vi "SPIM control3d-PID.vi"() -> ()   [LabVIEW 2012]
uses:
  Scanning Setting.vi
panel:
  in  "1 Slice":bool
  in  "Structual":bool
  in  "Funcational":bool
  out "Peizo Voltage":dbl
  out "Peizo Location":dbl
  out "Z-Offset":dbl
  out "Scan Signal 2":cluster{"Y":dbl[], "Y":dbl[]}[](graph)
  out "Trigger":dynamicdata(graph)=[{"t0"=timestamp(16448.7 s since 1904-01-01), "dt"=1e-05, "Y"=array[10000 elements], "attributes"=variant("NI_ChannelName"=variant(string "Triangle (Collected)"), "NI_ExpIsRelativeTime"=variant(bool TRUE), "NI_ExpStartTimeStamp"=variant(timestamp timestamp(3461934223.089551 s since 1904-01-01)), "NI_ExpTimeStamp"=variant(timestamp timestamp(3461934223.089551 s since 1904-01-01)), "NI_ExpXDimension"=variant(string "t"), "NI_OriginalChannelName"=variant(string "Triangle"))}, {"t0"=timestamp(16448.7 s since 1904-01-01), "dt"=1e-05, "Y"=array[10000 elements], "attributes"=variant("NI_ChannelName"=variant(string "Square (Collected)"), "NI_ExpIsRelativeTime"=variant(bool TRUE), "NI_ExpStartTimeStamp"=variant(timestamp timestamp(3461934223.089551 s since 1904-01-01)), "NI_ExpTimeStamp"=variant(timestamp timestamp(3461934223.089551 s since 1904-01-01)), "NI_ExpXDimension"=variant(string "t"), "NI_OriginalChannelName"=variant(string "Square"))}, {"t0"=timestamp(16448.7 s since 1904-01-01), "dt"=1e-05, "Y"=array[10000 elements], "attributes"=variant("NI_ChannelName"=variant(string "Square (Collected)"), "NI_ExpIsRelativeTime"=variant(bool TRUE), "NI_ExpStartTimeStamp"=variant(timestamp timestamp(3461934223.0885506 s since 1904-01-01)), "NI_ExpTimeStamp"=variant(timestamp timestamp(3461934223.0885506 s since 1904-01-01)), "NI_ExpXDimension"=variant(string "t"), "NI_OriginalChannelName"=variant(string "Square"))}]
  out "Scan Signal":cluster{"Y":dbl[], "Y":dbl[]}[](graph)
  out "Error Out":errorcluster={"status"=TRUE, "code"=-200561, "source"="SPIM control.vi:Instance:14:1<append>\n<B>Data: </B>-10.007205\n<B>Specified Range Minimum: </B>-10.0\n<B>Specified Range Maximum: </B> 10.0\n\n<B>Task Name: </B>_unnamedTask<30>"}
  in  "Scanner":bool
  in  "Setting":bool
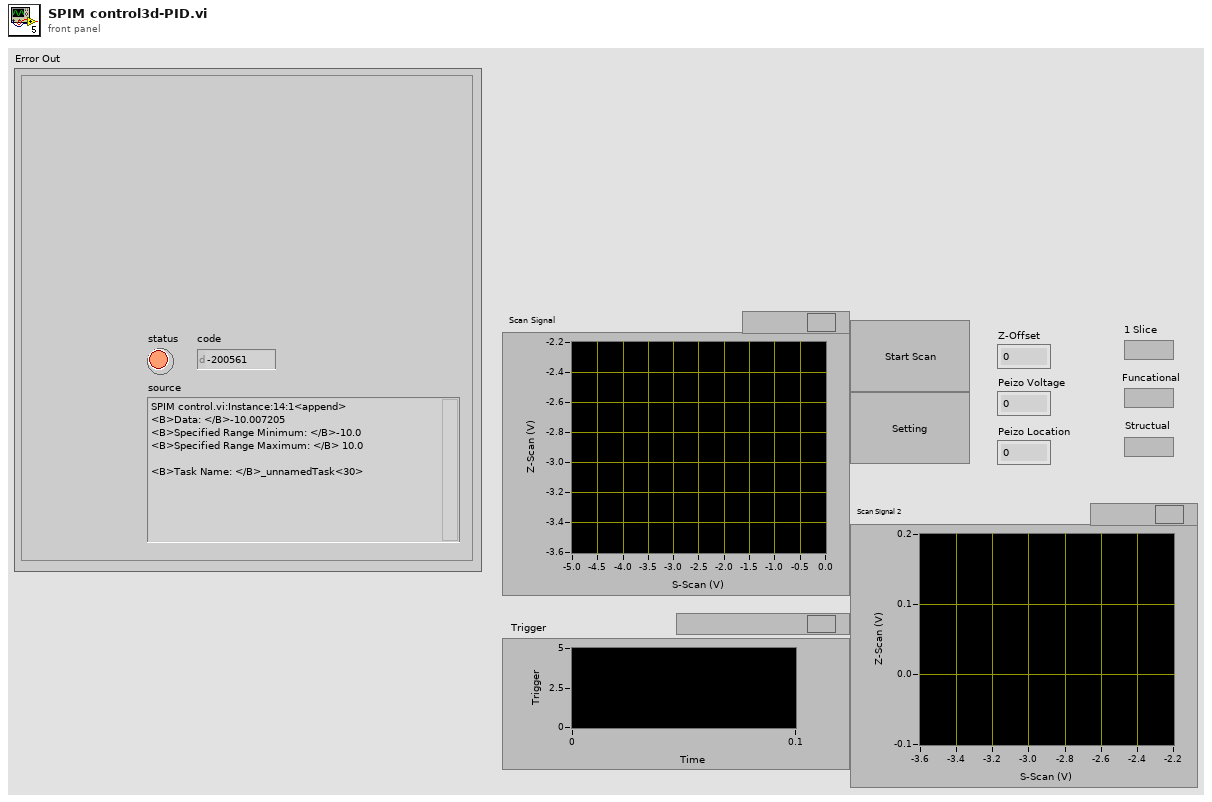
[diagram p1: front panel]
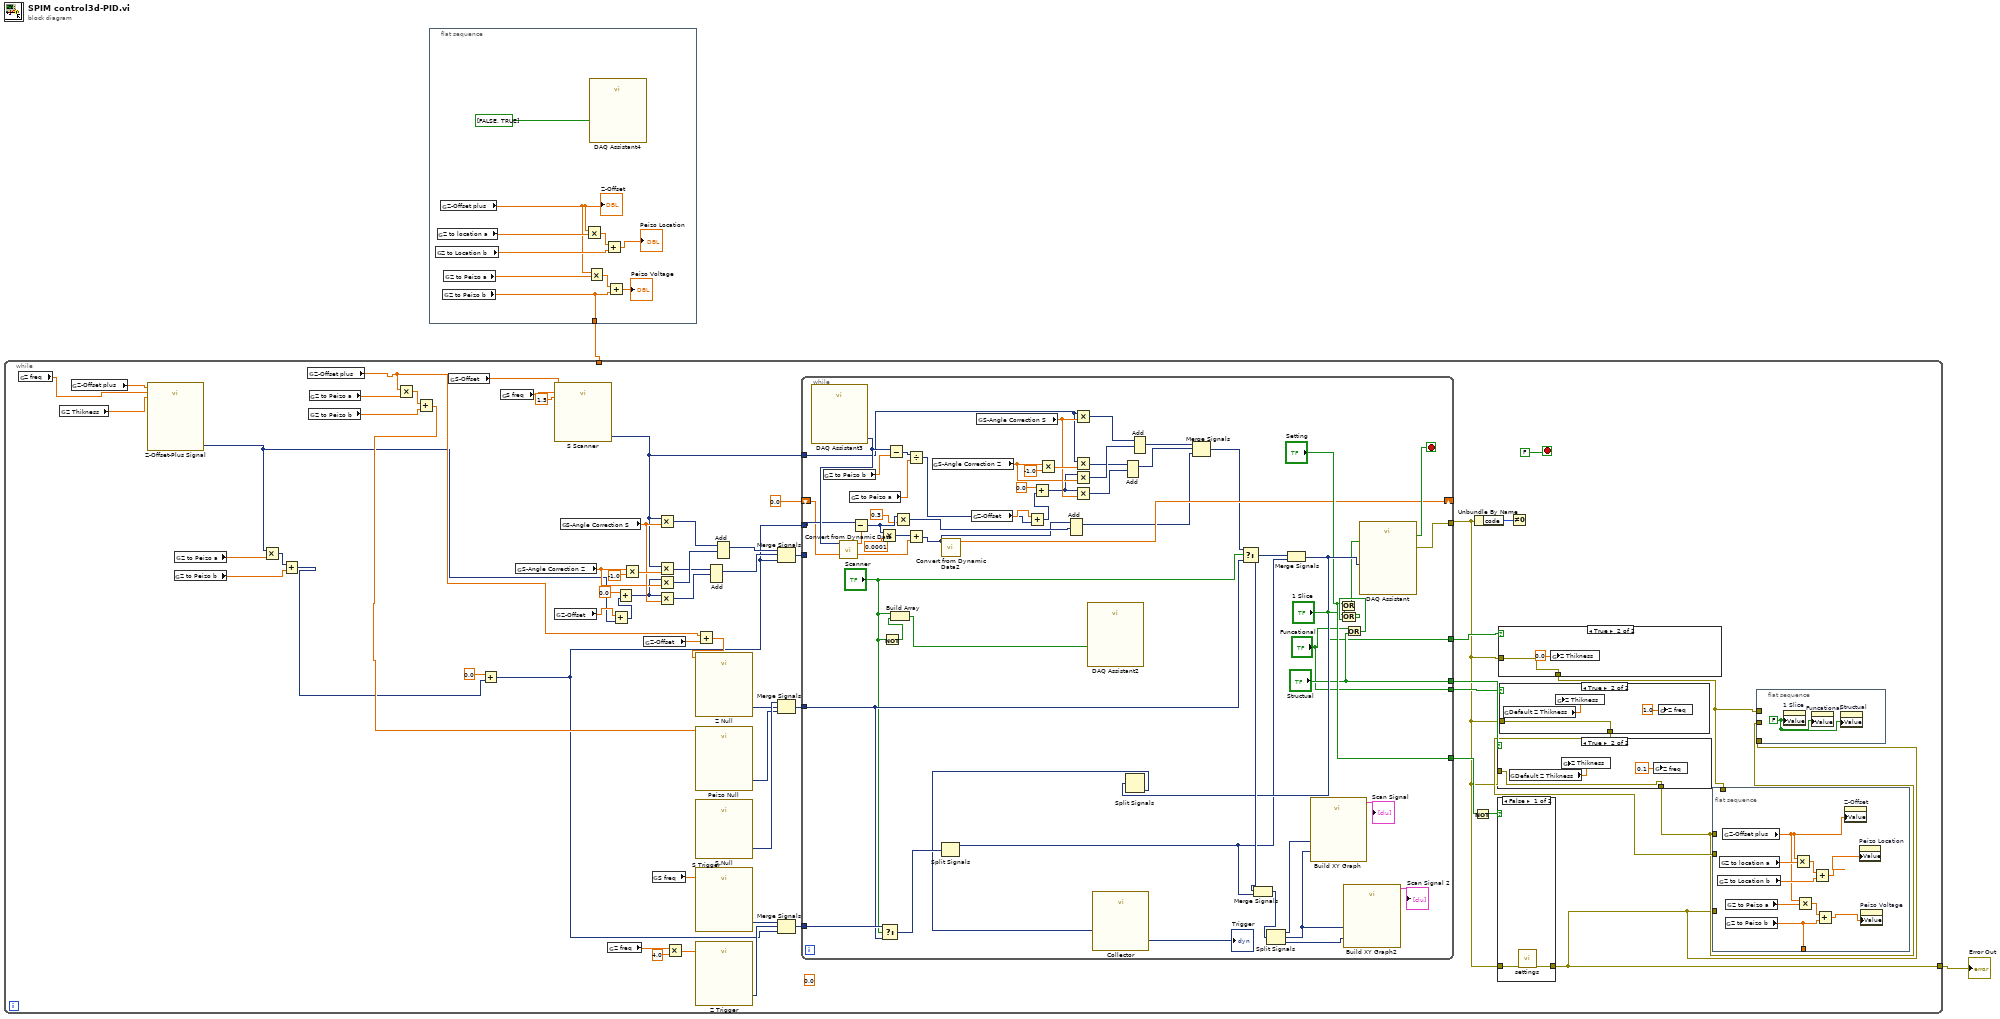
[diagram p0: block diagram]
diagram:
  n1 = while {
    tunnel: [w10] -> w1
    tunnel: w2 -> [_]
    stop <- FALSE stop-if-true
    (unwired) 0.0 ("Offset")
    n2 = global read "Scanning Setting.vi" "Z freq"() -> (w19:dbl)
    n3 = global read "Scanning Setting.vi" "Z Thikness"() -> (w20:dbl)
    n4 = global read "Scanning Setting.vi" "Z-Offset plus"() -> (w26:dbl)
    n5 = call "Z-Offset-Plus Signal"("Offset"=w26, "Frequency"=w19, "Amplitude"=w20) -> ("Triangle"=w21:dynamicdata)  [unwired: 11 in, 1 out]
    n6 = global read "Scanning Setting.vi" "Z to Peizo b"() -> (w25:dbl)
    n7 = global read "Scanning Setting.vi" "Z to Peizo a"() -> (w24:dbl)
    n8 = Multiply(x=w21, y=w24) -> (x*y=w23:dynamicdata)
    n9 = Add(x=w23, y=w25) -> (x+y=w22:dynamicdata)
    n10 = global read "Scanning Setting.vi" "Z-Offset plus"() -> (w27:dbl)
    n11 = global read "Scanning Setting.vi" "Z to Peizo b"() -> (w29:dbl)
    n12 = global read "Scanning Setting.vi" "Z to Peizo a"() -> (w30:dbl)
    n13 = Multiply(x=w27, y=w30) -> (x*y=w31:dbl)
    n14 = Add(x=w31, y=w29) -> (x+y=w28:dbl)
    n15 = global read "Scanning Setting.vi" "S-Offset"() -> (w50:dbl)
    n16 = Add(x=0.0, y=w22) -> (x+y=w5:dynamicdata)
    n17 = global read "Scanning Setting.vi" "S freq"() -> (w51:dbl)
    n18 = global read "Scanning Setting.vi" "S-Angle Correction Z"() -> (w48:dbl)
    n19 = call "S Scanner"("Offset"=w50, "Frequency"=w51, "Amplitude"=1.5) -> ("Triangle"=w6:dynamicdata)  [unwired: 11 in, 1 out]
    n20 = global read "Scanning Setting.vi" "Z-Offset"() -> (w35:dbl)
    n21 = global read "Scanning Setting.vi" "S-Angle Correction S"() -> (w49:dbl)
    n22 = global read "Scanning Setting.vi" "Z freq"() -> (w39:dbl)
    n23 = Add(x=w35, y=w21) -> (x+y=w34:dynamicdata)
    n24 = Add(x=0.0, y=w34) -> (x+y=w37:dynamicdata)
    n25 = Multiply(x=w48, y=-1.0) -> (x*y=w54:dbl)
    n26 = global read "Scanning Setting.vi" "Z-Offset"() -> (w33:dbl)
    n27 = global read "Scanning Setting.vi" "S freq"() -> (w45:dbl)
    n28 = Multiply(x=w6, y=w49) -> (x*y=w57:dynamicdata)
    n29 = Multiply(x=w6, y=w54) -> (x*y=w55:dynamicdata)
    n30 = Multiply(x=w37, y=w48) -> (x*y=w58:dynamicdata)
    n31 = Multiply(x=w37, y=w49) -> (x*y=w56:dynamicdata)
    n32 = Multiply(x=w39, y=4.0) -> (x*y=w40:dbl)
    n33 = call "Peizo Null"("Offset"=w28) -> ("Square"=w36:dynamicdata)  [unwired: 13 in, 1 out]
    n34 = call "S Null"() -> ("Triangle"=w62:dynamicdata)  [unwired: 14 in, 1 out]
    n35 = call "S Trigger"("Frequency"=w45) -> ("Square"=w44:dynamicdata)  [unwired: 13 in, 1 out]
    n36 = call "Z Trigger"("Frequency"=w40) -> ("Square"=w43:dynamicdata)  [unwired: 13 in, 1 out]
    n37 = Add(x=w27, y=w33) -> (x+y=w32:dbl)
    n38 = call "Z Null"("Offset"=w32) -> ("Square"=w47:dynamicdata)  [unwired: 13 in, 1 out]
    n39 = Add(1:w56, 2:w55) -> (0:w52:dynamicdata)  [unwired: 1 in, 1 out]
    n40 = Add(1:w58, 2:w57) -> (0:w46:dynamicdata)  [unwired: 1 in, 1 out]
    n41 = Merge Signals(w46, w52, w5) -> (w61:dynamicdata)
    n42 = Merge Signals(w62, w47, w36) -> (w60:dynamicdata)
    n43 = Merge Signals(w44, w43, w5) -> (w42:dynamicdata)
    n44 = while {
      tunnel: w61 -> [_]
      tunnel: w60 -> [w138]
      tunnel: [w142] -> w9
      tunnel: w42 -> [w139]
      tunnel: ["Setting"] -> w17
      tunnel: ["Structual"] -> w16
      tunnel: ["Funcational"] -> w15
      tunnel: ["1 Slice"] -> w14
      tunnel: w6 -> [w87]
      tunnel: w5 -> [w99]
      shift-right: [w94] -> _
      shift-left: 0.0 ("x") -> [w95]
      stop <- w144 stop-if-true
      n45 = call "DAQ Assistant3"() -> ("data"=w100:dynamicdata)  [unwired: 16 in, 3 out]
      n46 = global read "Scanning Setting.vi" "Z to Peizo b"() -> (w118:dbl)
      n47 = call "Convert from Dynamic Data"("Dynamic Data Type"=w100) -> ("Scalar"=w98:dbl)  [unwired: 3 in]
      n48 = global read "Scanning Setting.vi" "Z to Peizo a"() -> (w116:dbl)
      n49 = Subtract(x=w99, y=w98) -> (x-y=w93:dynamicdata)
      n50 = Multiply(x=w93, y=0.0001) -> (x*y=w96:dynamicdata)
      n51 = Select(t=w139, s="Scanner", f=w138) -> (s? t:f=w133:dynamicdata)
      n52 = Not(x="Scanner") -> (.not. x?=w120:bool)
      n53 = Subtract(x=w100, y=w118) -> (x-y=w117:dynamicdata)
      n54 = Build Array("Scanner", w120) -> (w121:bool[])
      n55 = Multiply(x=w93, y=0.3) -> (x*y=w91:dynamicdata)
      n56 = Divide(x=w117, y=w116) -> (x/y=w103:dynamicdata)
      n57 = Add(x=w96, y=w95) -> (x+y=w90:dynamicdata)
      n58 = global read "Scanning Setting.vi" "S-Angle Correction Z"() -> (w108:dbl)
      n59 = Split Signals(w133) -> (w129:dynamicdata)  [unwired: 3 in, 2 out]
      n60 = call "Convert from Dynamic Data2"("Dynamic Data Type"=w90) -> ("Scalar"=w94:dbl)  [unwired: 3 in]
      n61 = global read "Scanning Setting.vi" "Z-Offset"() -> (w106:dbl)
      n62 = global read "Scanning Setting.vi" "S-Angle Correction S"() -> (w109:dbl)
      n63 = Add(x=w106, y=w103) -> (x+y=w105:dynamicdata)
      n64 = Add(x=0.0, y=w105) -> (x+y=w107:dynamicdata)
      n65 = Multiply(x=w108, y=-1.0) -> (x*y=w111:dbl)
      n66 = Add(1:w91, 2:w90) -> (0:w89:dynamicdata)  [unwired: 1 in, 1 out]
      n67 = Multiply(x=w87, y=w109) -> (x*y=w114:dynamicdata)
      n68 = Multiply(x=w87, y=w111) -> (x*y=w112:dynamicdata)
      n69 = Multiply(x=w107, y=w108) -> (x*y=w115:dynamicdata)
      n70 = Multiply(x=w107, y=w109) -> (x*y=w113:dynamicdata)
      n71 = call "DAQ Assistant2"("data"=w121) -> ()  [unwired: 17 in, 2 out]
      n72 = Add(1:w113, 2:w112) -> (0:w101:dynamicdata)  [unwired: 1 in, 1 out]
      n73 = Add(1:w115, 2:w114) -> (0:w102:dynamicdata)  [unwired: 1 in, 1 out]
      n74 = Merge Signals(w102, w101, w89) -> (w88:dynamicdata)
      n75 = Select(t=w88, s="Scanner", f=w138) -> (s? t:f=w141:dynamicdata)
      n76 = Merge Signals(w141, w129) -> (w130:dynamicdata)
      n77 = Split Signals(w130) -> (w135:dynamicdata, w136:dynamicdata, w134:dynamicdata)  [unwired: 3 in]
      n78 = Merge Signals(w141, w129) -> (w132:dynamicdata)
      n79 = Split Signals(w132) -> (w131:dynamicdata)  [unwired: 4 in, 3 out]
      n80 = call "Collector"("Signals"=w131) -> ("Collected Signals"=→"Trigger":dynamicdata)  [unwired: 9 in, 1 out]
      n81 = call "Build XY Graph"("Y Input"=w136, "X Input"=w135) -> ("XY Graph"=→"Scan Signal":cluster{"Y":dbl[], "Y":dbl[]}[])  [unwired: 3 in, 6 out]
      n82 = call "Build XY Graph2"("Y Input"=w134, "X Input"=w136) -> ("XY Graph"=→"Scan Signal 2":cluster{"Y":dbl[], "Y":dbl[]}[])  [unwired: 3 in, 6 out]
      n83 = Or(x="Funcational", y="Structual") -> (x .or. y?=w128:bool)
      n84 = Or(x="1 Slice", y=w128) -> (x .or. y?=w127:bool)
      n85 = Or(x="Setting", y=w127) -> (x .or. y?=w125:bool)
      n86 = call "DAQ Assistant"("data"=w132, "stop (F)"=w125) -> ("stopped"=w144:bool, "error out"=w142:errorcluster)  [unwired: 15 in, 1 out]
    }
    n87 = Not(x=w17) -> (.not. x?=w18:bool)
    n88 = Unbundle By Name(w9) -> ("code"=w38:i32)
    n89 = case shown="True" w16 {
      tunnel: w9 -> [w71 w72]
      tunnel: [w71 w72] -> w11
      frame False {
      }
      frame True {
        n90 = global read "Scanning Setting.vi" "Default Z Thikness"() -> (w74:dbl)
        n91 = global write "Scanning Setting.vi" "Z Thikness"(w74) -> ()
        n92 = global write "Scanning Setting.vi" "Z freq"(0.1 ("Z freq")) -> ()
      }
    }
    n93 = case shown="False" w18 {
      tunnel: [w84 w86] -> w10
      tunnel: w9 -> [w85 w86]
      frame False {
        n94 = call "settings.vi"("Error In"=w85) -> ("Error Out"=w84:errorcluster)  [unwired: 10 in]
      }
      frame True {
      }
    }
    n95 = case shown="True" w14 {
      tunnel: w9 -> [w64 w65]
      tunnel: [w64 w65] -> w12
      frame False {
      }
      frame True {
        n96 = global write "Scanning Setting.vi" "Z Thikness"(0.0 ("Z Thikness")) -> ()
      }
    }
    n97 = case shown="True" w15 {
      tunnel: w9 -> [w67 w68]
      tunnel: [w67 w68] -> w13
      frame False {
      }
      frame True {
        n98 = global read "Scanning Setting.vi" "Default Z Thikness"() -> (w70:dbl)
        n99 = global write "Scanning Setting.vi" "Z Thikness"(w70) -> ()
        n100 = global write "Scanning Setting.vi" "Z freq"(1.0 ("Z freq")) -> ()
      }
    }
    n101 = Not Equal To 0?(x=w38) -> ()  [unwired: 1 out]
    n102 = flat-sequence {
      tunnel: [w78] -> _
      tunnel: w10 -> [_]
      tunnel: w11 -> [_]
      tunnel: w13 -> [_]
      tunnel: w12 -> [_]
      frame #0 {
        n103 = global read "Scanning Setting.vi" "Z to Location b"() -> (w81:dbl)
        n104 = global read "Scanning Setting.vi" "Z to location a"() -> (w83:dbl)
        n105 = global read "Scanning Setting.vi" "Z-Offset plus"() -> (w77:dbl)
        n106 = global read "Scanning Setting.vi" "Z to Peizo b"() -> (w78:dbl)
        n107 = global read "Scanning Setting.vi" "Z to Peizo a"() -> (w79:dbl)
        n108 = Multiply(x=w77, y=w83) -> (x*y=w82:dbl)
        n109 = Multiply(x=w77, y=w79) -> (x*y=w80:dbl)
        n110 = Add(x=w82, y=w81) -> (x+y=w76:dbl)
        n111 = Add(x=w80, y=w78) -> (x+y=w75:dbl)
        n112 = property on="Z-Offset" class="DigNum (strict)"("Value"=w77) -> ()  [unwired: 2 in, 2 out]
        n113 = property on="Peizo Location" class="DigNum (strict)"("Value"=w76) -> ()  [unwired: 2 in, 2 out]
        n114 = property on="Peizo Voltage" class="DigNum (strict)"("Value"=w75) -> ()  [unwired: 2 in, 2 out]
      }
    }
    n115 = flat-sequence {
      tunnel: w12 -> [_]
      tunnel: w11 -> [_]
      tunnel: w10 -> [_]
      frame #0 {
        w63 = FALSE ("1 Slice")
        n116 = property on="1 Slice" class="Bool (strict)"("Value"=w63) -> ()  [unwired: 2 in, 2 out]
        n117 = property on="Funcational" class="Bool (strict)"("Value"=w63) -> ()  [unwired: 2 in, 2 out]
        n118 = property on="Structual" class="Bool (strict)"("Value"=w63) -> ()  [unwired: 2 in, 2 out]
      }
    }
  }
  "Error Out" <- w1
  n119 = flat-sequence {
    tunnel: [w146] -> w2
    frame #0 {
      n120 = global read "Scanning Setting.vi" "Z to Location b"() -> (w152:dbl)
      n121 = global read "Scanning Setting.vi" "Z to location a"() -> (w154:dbl)
      n122 = global read "Scanning Setting.vi" "Z-Offset plus"() -> (w147:dbl)
      "Z-Offset" <- w147
      n123 = global read "Scanning Setting.vi" "Z to Peizo b"() -> (w146:dbl)
      n124 = global read "Scanning Setting.vi" "Z to Peizo a"() -> (w149:dbl)
      n125 = Multiply(x=w147, y=w154) -> (x*y=w153:dbl)
      n126 = Multiply(x=w147, y=w149) -> (x*y=w150:dbl)
      n127 = call "DAQ Assistant4"("data"=bool[] [FALSE, TRUE]) -> ()  [unwired: 17 in, 2 out]
      n128 = Add(x=w153, y=w152) -> (x+y=→"Peizo Location":dbl)
      n129 = Add(x=w150, y=w146) -> (x+y=→"Peizo Voltage":dbl)
    }
  }
